vi "Parse-attribute.vi"(8 "error in (no error)":errorcluster, 10 "String in":string, 11 "LaserEnableDelay in":refnum<class "LaserEnableDelay.lvclass">) -> (0 "error out":errorcluster, 1 "Valid attribute?":bool, 2 "Remaining string":string, 3 "LaserEnableDelay out":refnum<class "LaserEnableDelay.lvclass">)   [LabVIEW 2013, in "MaterialCharacterization.lvlib" / "LaserEnableDelay.lvclass"]
uses:
  LaserEnableDelay.lvclass
  Attributes.ctl
  Attribute-ID.ctl
  Attribute-XML.lvclass/Attribute-XML.ctl
  ID.lvclass/ID.ctl
  Time/Time.lvclass/Time.ctl
  Write Attribute.vi
  Write ID-attribute.vi
  Time/Write Time interval.vi
  Attribute-XML.lvclass
  ID.lvclass
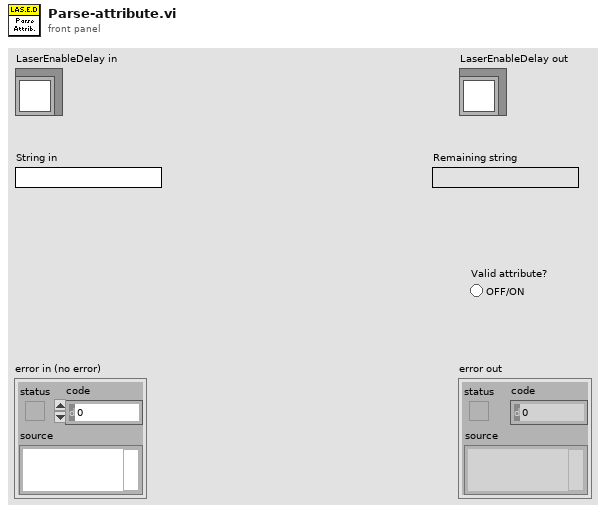
[diagram p1: front panel]
types:
  T1 = typedef "MaterialCharacterization.lvlib/ID.lvclass/Attribute-ID.ctl" = enum16{"FieldOffset", "TransformEnable", "Transform", "Units", "XYCalFactor", "EnableLaser", "JumpDelay", "MarkDelay", "PolyDelay", "LaserOnDelay", "LaserOffDelay", "JumpSpeed", "MarkSpeed", "LaserPowerDelay", "LaserEnableDelay", "LaserPower", "Offset"}
  T2 = typedef "MaterialCharacterization.lvlib/Attribute-XML.lvclass/Attributes.ctl" = enum16{"id"}
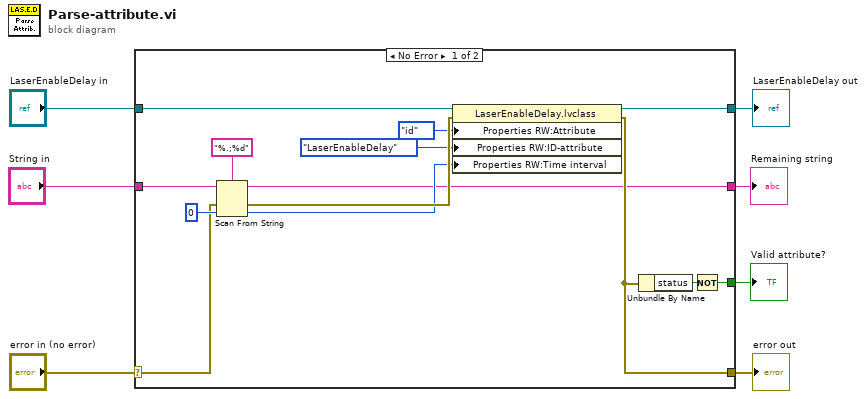
[diagram p0: block diagram]
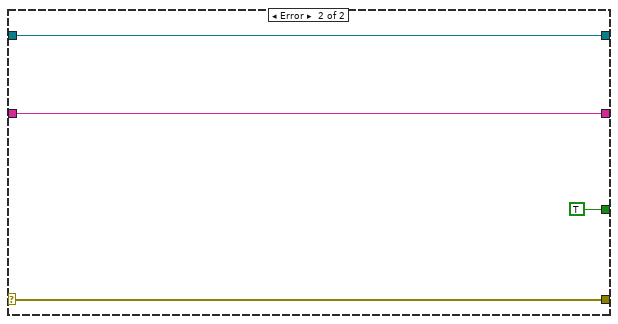
[diagram p2: hidden frame]
diagram:
  n1 = case shown="No Error" "error in (no error)" {
    selector: "error in (no error)" -> [w13 w25]
    tunnel: [w12 w25] -> w6
    tunnel: [w8 w24] -> w4
    tunnel: "LaserEnableDelay in" -> [w9 w24]
    tunnel: "String in" -> [w14 w23]
    tunnel: [w11 TRUE] -> w2
    tunnel: [w10 w23] -> w1
    frame No Error {
      n2 = Scan From String(format string="%.;%d", input string=w14, error in=w13, default 1=i64 0 ("default value 2")) -> (remaining string=w10:string, error out=w19:errorcluster, output 1=w16:i64)  [unwired: 1 in, 1 out]
      n3 = property class="LaserEnableDelay.lvclass"(reference=w9, error in=w19, "Properties RW:Attribute"=Attributes."id" ("Attribute"), "Properties RW:ID-attribute"=Attribute-ID."LaserEnableDelay" ("ID-attribute"), "Properties RW:Time interval"=w16) -> (reference out=w8:refnum<class "LaserEnableDelay.lvclass">, error out=w12:errorcluster)
      n4 = Unbundle By Name(w12) -> ("status"=w20:bool)
      n5 = Not(x=w20) -> (.not. x?=w11:bool)
    }
    frame Error {
    }
  }
  "error out" <- w6
  "LaserEnableDelay out" <- w4
  "Remaining string" <- w1
  "Valid attribute?" <- w2
